vi "PQuntrace.vi"(8 "error in (no error)":errorcluster) -> (0 "error out":errorcluster)   [LabVIEW 2019, in "libpqlv.lvlib"]
uses:
  libpqlv.lvlib
  libpq.dll
panel:
  in  "conn":u32
  out "conn_out":u32
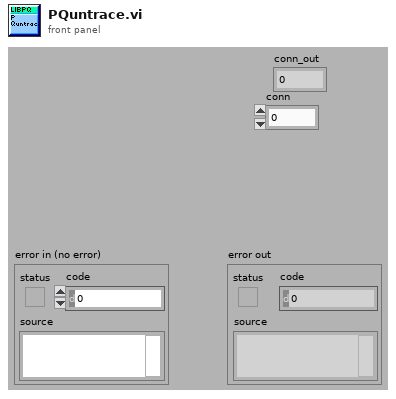
[diagram p1: front panel]
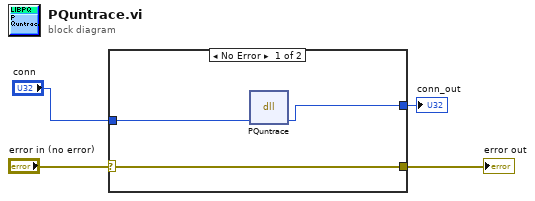
[diagram p0: block diagram]
diagram:
  n1 = case shown="No Error" "error in (no error)" {
    selector: "error in (no error)" -> [w7 w9]
    tunnel: [w7 w9] -> w3
    tunnel: [w6 w8] -> w2
    tunnel: "conn" -> [w5 w8]
    frame No Error {
      n2 = dll-call lib="libpq.*" fn="PQuntrace"("conn"=w5) -> ("conn"=w6:u32)  [unwired: 4 in, 2 out]
    }
    frame Error {
    }
  }
  "error out" <- w3
  "conn_out" <- w2
